vi "Update Analysis 1D U16.vi"(8 "error in (no error)":errorcluster, 9 "Image Series":u16[](array[numeric]), 10 "Analysis Image":dbl[][](array[numeric]), 11 "Analysis Graph in":refnum<class "Analysis Graph.lvclass">) -> (0 "error out":errorcluster, 1 "pixel signal roied  out":u16[](array[numeric]), 2 "Cursor.Cursor Position":T1, 3 "Analysis Graph out":refnum<class "Analysis Graph.lvclass">)   [LabVIEW 2023, in "Analysis Graph.lvclass"]
uses:
  Analysis Graph.lvclass
  D:/git/Graph-Classes/graph-classes/Detail Graph/Detail Graph.lvclass
  D:/git/Graph-Classes/graph-classes/Series Graph/Series Graph.lvclass
  <vilib>/Utility/miscctls.llb/LVPointDoubleTypeDef.ctl
  Analysis Graph.lvclass/Analysis Graph.ctl
  Detail Graph/Detail Graph.lvclass
  Series Graph/Series Graph.lvclass
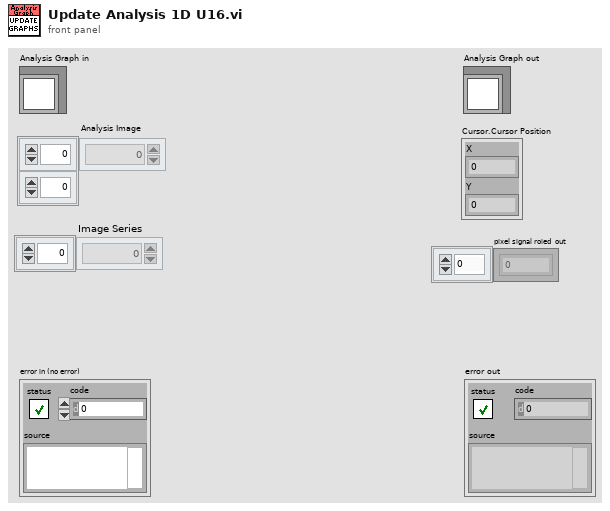
[diagram p1: front panel]
types:
  T1 = typedef "LVPointDoubleTypeDef.ctl" = cluster{"X":dbl, "Y":dbl}
  T2 = cluster{"ROI X":cluster{"Index":u32, "Length":u32}, "ROI Y":cluster{"Index":u32, "Length":u32}, "ROI Z":cluster{"Index":u32, "Length":u32}}
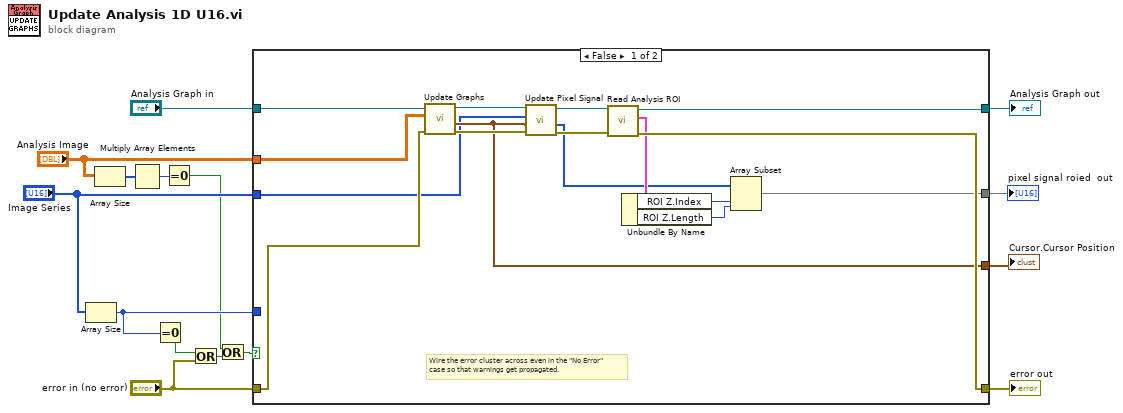
[diagram p0: block diagram]
diagram:
  n1 = Array Size(array="Image Series") -> (size(s)=w10:i32)
  n2 = Array Size(array="Analysis Image") -> (size(s)=w5:i32[])
  n3 = Multiply Array Elements(1:w5) -> (0:w4:i32)
  n4 = Equal To 0?(x=w10) -> (x = 0?=w12:bool)
  n5 = Equal To 0?(x=w4) -> (x = 0?=w3:bool)
  n6 = Or(x=w12, y="error in (no error)") -> (x .or. y?=w2:bool)
  n7 = Or(x=w3, y=w2) -> (x .or. y?=w1:bool)
  n8 = case shown="False" w1 {
    tunnel: [w30 w32] -> w15
    tunnel: [w27 w33] -> w13
    tunnel: "Analysis Graph in" -> [w29 w33]
    tunnel: "error in (no error)" -> [w28 w32]
    tunnel: w10 -> [_ _]
    tunnel: "Analysis Image" -> [w31 _]
    tunnel: "Image Series" -> [w21 _]
    tunnel: [w22 _] -> w8
    tunnel: [w17 _] -> w7
    frame False {
      # "Wire the error cluster across even in the \"No Error\"\ncase so that warnings get propagated."
      n9 = call "Update Graphs.vi"("error in (no error)"=w28, "image"=w31, "Detail Graph in"=w29) -> ("error out"=w24:errorcluster, "Cursor.Cursor Position"=w22:T1, "Detail Graph out"=w26:refnum<class "Analysis Graph.lvclass">)  [unwired: 6 in]
      n10 = call "Update Pixel Signal.vi"("error in (no error)"=w24, "Cursor.Cursor Position"=w22, "Image Series"=w21, "Series Graph in"=w26) -> ("error out"=w23:errorcluster, "Image Series  out"=w16:u16[], "Series Graph out"=w25:refnum<class "Analysis Graph.lvclass">)  [unwired: 5 in]
      n11 = call "Read Analysis ROI.vi"("error in (no error)"=w23, "Analysis Graph in"=w25) -> ("error out"=w30:errorcluster, "ROI XYZ"=w20:T2, "Analysis Graph out"=w27:refnum<class "Analysis Graph.lvclass">)  [unwired: 7 in]
      n12 = Unbundle By Name(w20) -> ("ROI Z.Index"=w19:u32, "ROI Z.Length"=w18:u32)
      n13 = Array Subset(array=w16, index=w19, length=w18) -> (w17:u16[])
    }
    frame True {
    }
  }
  "error out" <- w15
  "Analysis Graph out" <- w13
  "Cursor.Cursor Position" <- w8
  "pixel signal roied  out" <- w7
